vi "NoErrorRead.vi"(8 "error in":errorcluster, 10 "MessageBuffer":T1, 11 "Channel":u16) -> (0 "error out":errorcluster, 2 "MessageBuffer out":T1, 3 "Channel out":u16, 5 "function return":u32)   [LabVIEW 2025, in "PCAN API.lvlib"]
doc: "This VI is used for writting a CAN message without decoding errors from function return."
uses:
  PCAN API.lvlib
  PCAN2023/PCAN2023.lvlib
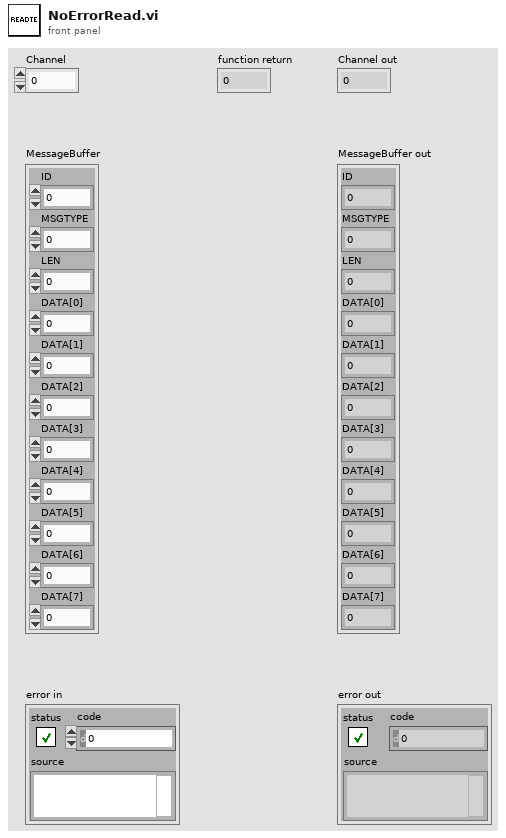
[diagram p1: front panel]
types:
  T1 = cluster{"ID":u32, "MSGTYPE":u8, "LEN":u8, "DATA[0]":u8, "DATA[1]":u8, "DATA[2]":u8, "DATA[3]":u8, "DATA[4]":u8, "DATA[5]":u8, "DATA[6]":u8, "DATA[7]":u8}
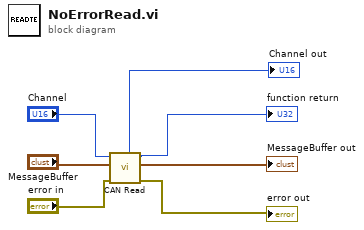
[diagram p0: block diagram]
diagram:
  n1 = call "CAN Read.vi"("error in"="error in", "MessageBuffer"="MessageBuffer", "Channel"="Channel") -> ("error out"=→"error out":errorcluster, "MessageBuffer out"=→"MessageBuffer out":T1, "function return"=→"function return":u32, "Channel out"=→"Channel out":u16)  [unwired: 4 in, 1 out]
